vi "sigmoid.vi"(7 "Input":dbl[](array[numeric]), 11 "Derivative?":bool) -> (6 "Output":dbl[](array[numeric]))   [LabVIEW 2016]
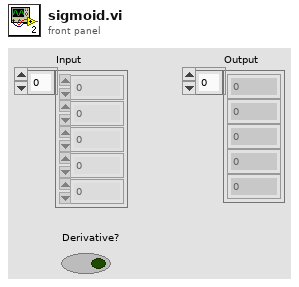
[diagram p1: front panel]
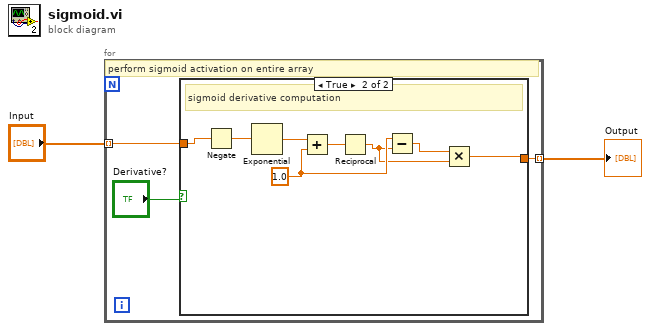
[diagram p0: block diagram]
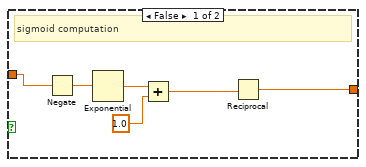
[diagram p2: hidden frame]
diagram:
  n1 = for {
    tunnel: "Input" -> [w5] mode=indexing
    tunnel: [w4] -> w1 mode=indexing
    # "perform sigmoid activation on entire array"
    n2 = case shown="True" "Derivative?" {
      tunnel: w5 -> [w10 w17]
      tunnel: [w11 w12] -> w4
      frame False {
        # "sigmoid computation"
        n3 = Negate(x=w10) -> (-x=w9:dbl)
        n4 = Exponential(1:w9) -> (0:w8:dbl)
        n5 = Add(x=w8, y=1.0) -> (x+y=w6:dbl)
        n6 = Reciprocal(x=w6) -> (1/x=w11:dbl)
      }
      frame True {
        w15 = 1.0
        # "sigmoid derivative computation"
        n7 = Negate(x=w17) -> (-x=w19:dbl)
        n8 = Exponential(1:w19) -> (0:w18:dbl)
        n9 = Add(x=w18, y=w15) -> (x+y=w16:dbl)
        n10 = Reciprocal(x=w16) -> (1/x=w13:dbl)
        n11 = Subtract(x=w15, y=w13) -> (x-y=w14:dbl)
        n12 = Multiply(x=w14, y=w13) -> (x*y=w12:dbl)
      }
    }
  }
  "Output" <- w1
